vi "Write U8 To 1 Address.vi"(0 "VISA resource name":refnum<visa-resource-name>, 5 "Motor ID (0)":u8, 7 "Address number (0)":u8, 9 "Parameter (0)":u8, 11 "error in (no error)":errorcluster) -> (4 "VISA resource name out":refnum<visa-resource-name>, 15 "error out":errorcluster)   [LabVIEW 2016, in "Dynamixel Motor.lvlib"]
doc: "Writes a U8 to one address of the register on the motor. This is a Low-Level VI that is used by other VIs."
uses:
  Dynamixel Motor.lvlib
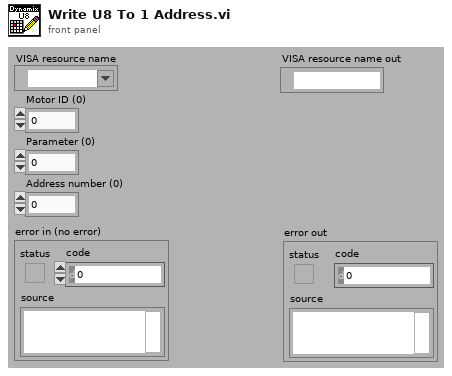
[diagram p1: front panel]
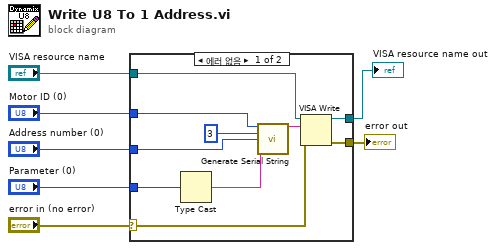
[diagram p0: block diagram]
diagram:
  n1 = case shown="에러 없음" "error in (no error)" {
    selector: "error in (no error)" -> [w13 w19]
    tunnel: "Parameter (0)" -> [w9 _]
    tunnel: "Address number (0)" -> [w10 _]
    tunnel: "Motor ID (0)" -> [w12 _]
    tunnel: "VISA resource name" -> [w17 w18]
    tunnel: [w15 w19] -> w3
    tunnel: [w14 w18] -> w2
    frame No Error {
      n2 = Type Cast(x=w9) -> (*(type *) &x=w8:string)  [unwired: 1 in]
      n3 = call "Generate Serial String.vi"("Motor ID"=w12, "Command"=u8 3, "Address"=w10, "Parameters"=w8) -> ("Command to Serial"=w16:string)  [unwired: 10 in, 1 out]
      n4 = VISA Write(VISA resource name=w17, write buffer=w16, error in (no error)=w13) -> (VISA resource name out=w14:refnum<visa-resource-name>, error out=w15:errorcluster)  [unwired: 1 out]
    }
    frame Error {
    }
  }
  "error out" <- w3
  "VISA resource name out" <- w2
